vi "Read Transfer Group Buffer.vi"(8 "error in (no error)":errorcluster, 10 "Transfer Group":refnum<class "Transfer Group.lvclass">, 11 "UDP Transceiver in":refnum<class "UDP Transceiver.lvclass">) -> (0 "error out":errorcluster, 1 "data":string, 3 "UDP Transceiver out":refnum<class "UDP Transceiver.lvclass">)   [LabVIEW 2017, in "UDP.lvlib" / "UDP Transceiver.lvclass"]
uses:
  UDP Transceiver.lvclass
  DSF Core.lvlibp/Classes/Transfer Group/Transfer Group.lvclass
  UDP Transceiver.lvclass/UDP Transceiver.ctl
  DSF Core.lvlibp/Classes/Buffer/Read Buffer 1D U8.vi
  DSF Core.lvlibp/Classes/Buffer/Buffer.lvclass
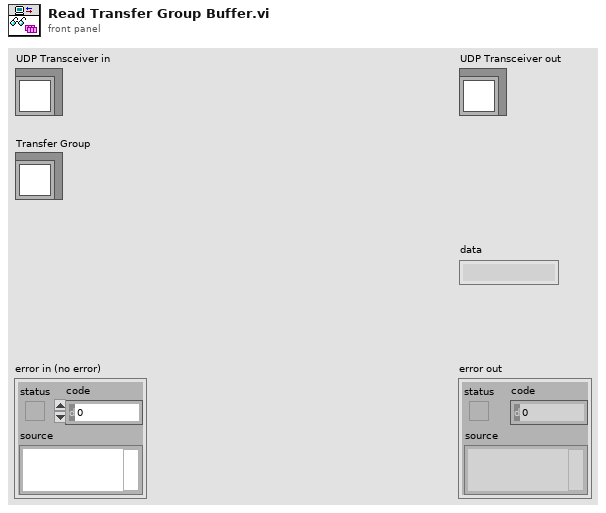
[diagram p1: front panel]
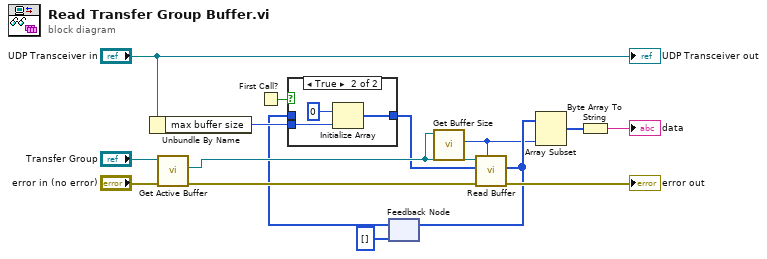
[diagram p0: block diagram]
diagram:
  n1 = Unbundle By Name("UDP Transceiver in") -> ("max buffer size"=w6:u64)
  n2 = call "Get Active Buffer.vi"("error in (no error)"="error in (no error)", "Transfer Group in"="Transfer Group") -> ("error out"=w11:errorcluster, "Buffer"=w5:refnum<class "Buffer.lvclass">)  [unwired: 7 in, 1 out]
  n3 = First Call?() -> (First Call?: T/F=w7:bool)
  n4 = feedback #1(u8[] []) -> (w3:u8[])
  n5 = case shown="True" w7 {
    tunnel: w3 -> [w16 _]
    tunnel: [w16 w19] -> w4
    tunnel: w6 -> [_ w17]
    frame False {
    }
    frame True {
      n6 = Initialize Array(u8 0 ("Numeric"), w17) -> (w19:u8[])
    }
  }
  n7 = call "Get Buffer Size.vi"("Buffer in"=w5) -> ("buffer size"=w1:u64)  [unwired: 9 in, 1 out]
  n8 = call-poly "Read Buffer.vi"("count (-1: rest)"=w1, "error in (no error)"=w11, "dst array in"=w4, "Buffer in"=w5) -> ("error out"=→"error out":errorcluster, "dst array out"=w2:u8[])  [unwired: 4 in, 2 out]
  n9 = feedback-in #1(w2) -> ()
  n10 = Array Subset(array=w2, length=w1) -> (w13:u8[])  [unwired: 1 in]
  n11 = Byte Array To String(unsigned byte array=w13) -> (string=→"data":string)
  "UDP Transceiver out" <- "UDP Transceiver in"
